vi "SingleMeasurement.vi"(8 "error in (no error)":errorcluster, 11 "VISA resource name":refnum<visa-resource-name>) -> (0 "error out":errorcluster, 2 "output / s":dbl, 3 "VISA resource name out":refnum<visa-resource-name>)   [LabVIEW 2014, in "GP22_TDC_Arduinoed.lvlib"]
doc: "Take a single TDC measurement.\n\nIf the GP22 is not set to automatically calibrate on every run, perform a TDC calibration before the measurement."
uses:
  GP22_TDC_Arduinoed.lvlib
  Globals.vi
  Private/ConvertTimes - Single.vi
panel:
  out "read buffer":string
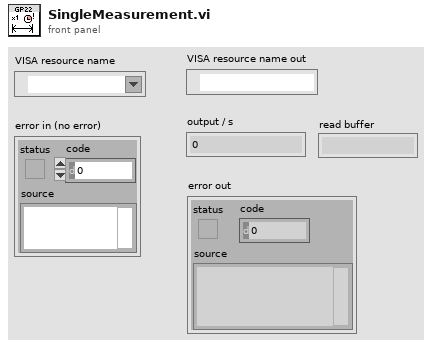
[diagram p1: front panel]
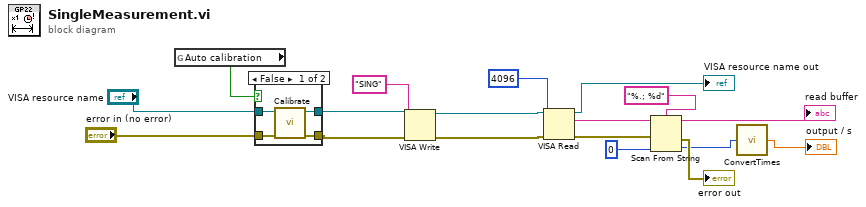
[diagram p0: block diagram]
diagram:
  n1 = global read "Globals.vi" "Auto calibration"() -> (w7:bool)
  n2 = case shown="False" w7 {
    tunnel: "VISA resource name" -> [w21 w23]
    tunnel: "error in (no error)" -> [w20 w22]
    tunnel: [w19 w22] -> w6
    tunnel: [w18 w23] -> w3
    frame False {
      n3 = call "Calibrate.vi"("error in (no error)"=w20, "VISA resource name"=w21) -> ("error out"=w19:errorcluster, "VISA resource name out"=w18:refnum<visa-resource-name>)  [unwired: 5 in, 2 out]
    }
    frame True {
    }
  }
  n4 = VISA Write(VISA resource name=w3, write buffer="SING" ("command"), error in (no error)=w6) -> (VISA resource name out=w2:refnum<visa-resource-name>, error out=w1:errorcluster)  [unwired: 1 out]
  n5 = VISA Read(VISA resource name=w2, byte count=u32 4096, error in (no error)=w1) -> (VISA resource name out=→"VISA resource name out":refnum<visa-resource-name>, read buffer=w14:string, error out=w13:errorcluster)  [unwired: 1 out]
  "read buffer" <- w14
  n6 = Scan From String(format string="%.; %d", input string=w14, error in=w13, default 1=u32 0 ("default value 1")) -> (error out=→"error out":errorcluster, output 1=w10:u32)  [unwired: 1 in, 2 out]
  n7 = call-poly "ConvertTimes.vi"("GP22 Output"=w10) -> ("Time/s"=→"output / s":dbl)
